vi "Volts to I16 - ARRAY.vi"(7 "Voltage (V)":dbl[](array[numeric])) -> (8 "I16":i16[](array[numeric]))   [LabVIEW 2014]
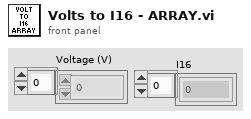
[diagram p1: front panel]
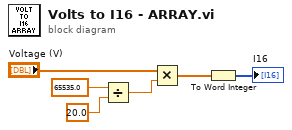
[diagram p0: block diagram]
diagram:
  n1 = Divide(x=65535.0, y=20.0 ("x")) -> (x/y=w4:dbl)
  n2 = Multiply(x="Voltage (V)", y=w4) -> (x*y=w3:dbl[])
  n3 = To Word Integer(number=w3) -> (16bit integer=→"I16":i16[])
